vi "FlattenedData1Darray to 2Darray.vi"(7 "Flattened data 1D array":T1[](array[typedef])) -> (3 "2D array":dbl[][](array[numeric]))   [LabVIEW 2017, in "SignalConverson.lvlib"]
uses:
  SignalConverson.lvlib
  FlattenedData.ctl
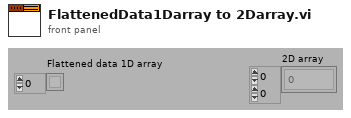
[diagram p1: front panel]
types:
  T1 = typedef "SignalConverson.lvlib/FlattenedData.ctl" = cluster{"V_A' [V]":dbl, "V_D' [V]":dbl, "V_P'  [V]":dbl, "V_S' [V]":dbl, "V_L' [V]":dbl, "V_R' [V]":dbl, "V_sum' [V]":dbl, "V_x [V]":dbl, "V_y [V]":dbl, "V_px' [V]":dbl, "V_py' [V]":dbl, "V_pz' [V]":dbl, "dt [s]":dbl, "Vpx_AO [V]":dbl, "Vpy_AO [V]":dbl, "Vpz_AO [V]":dbl, "scan backlog":dbl, "Counter":dbl, "TrapX [nm]":dbl, "TrapY [nm]":dbl, "TrapZ [nm]":dbl, "V_A [V]":dbl, "V_D [V]":dbl, "V_P [V]":dbl, "V_S [V]":dbl, "V_L [V]":dbl, "V_R [V]":dbl, "V_sum [V]":dbl, "V_x [V]":dbl, "V_y [V]":dbl, "P power [mW]":dbl, "S power [mW]":dbl, "angle compensated P power [W]":dbl, "angle compensated S power [W]":dbl, "angle compensated V_L":dbl, "angle compensated V_R":dbl, "angle compensated V_sum [V]":dbl, "angle compensated V_x [V]":dbl, "angle compensated V_y [V]":dbl, "Psi [rad]":dbl, "Laser power before objective[W]":dbl, "E_in":dbl, "E_out":dbl, "Delta E":dbl, "X signal":dbl, "Y signal":dbl, "Z signal":dbl, "TrapX (AO) [nm]":dbl, "TrapY (AO) [nm]":dbl, "TrapZ (AO) [nm]":dbl, "Fz [pN]":dbl, "Zext [nm]":dbl, "Tau [pNnm]":dbl, "Turn":dbl, "Fx [pN]":dbl, "Xext [nm]":dbl, "Fy [pN]":dbl, "Yext [nm]":dbl, "time [s]":dbl, "Delta Z signal":dbl, "Delta Z bead [nm]":dbl, "Z bead [nm]":dbl, "Delta TrapZ [nm]":dbl, "Delta Xsignal":dbl, "X bead [nm]":dbl, "Delta Ysignal":dbl, "Y bead [nm]":dbl, "Stop Condition":dbl}
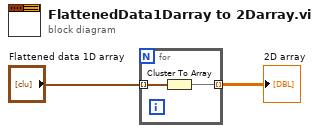
[diagram p0: block diagram]
diagram:
  n1 = for {
    tunnel: "Flattened data 1D array" -> [w4] mode=indexing
    tunnel: [w3] -> w1 mode=indexing
    n2 = Cluster To Array(cluster=w4) -> (array=w3:dbl[])
  }
  "2D array" <- w1
